vi "Read State.vi"(8 "error in (no error)":errorcluster, 11 "HECR in":refnum<class "PL SMC HECR.lvclass">) -> (0 "error out":errorcluster, 2 "state":T1, 3 "HECR out":refnum<class "PL SMC HECR.lvclass">)   [LabVIEW 2015, in "PL SMC HECR.lvclass"]
doc: "Reads device state."
uses:
  PL SMC HECR.lvclass
  <vilib>/plasmapper/PL Modbus Client/PL Modbus Client.lvclass
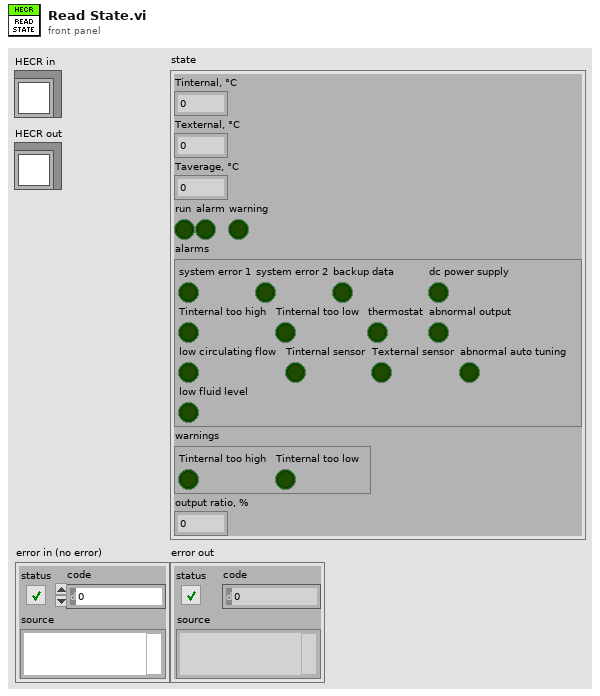
[diagram p1: front panel]
types:
  T1 = cluster{"Tinternal, °C":dbl, "Texternal, °C":dbl, "Taverage, °C":dbl, "run":bool, "alarm":bool, "warning":bool, "alarms":cluster{"system error 1":bool, "system error 2":bool, "backup data":bool, "dc power supply":bool, "Tinternal too high":bool, "Tinternal too low":bool, "thermostat":bool, "abnormal output":bool, "low circulating flow":bool, "Tinternal sensor":bool, "Texternal sensor":bool, "abnormal auto tuning":bool, "low fluid level":bool}, "warnings":cluster{"Tinternal too high":bool, "Tinternal too low":bool}, "output ratio, %":dbl}
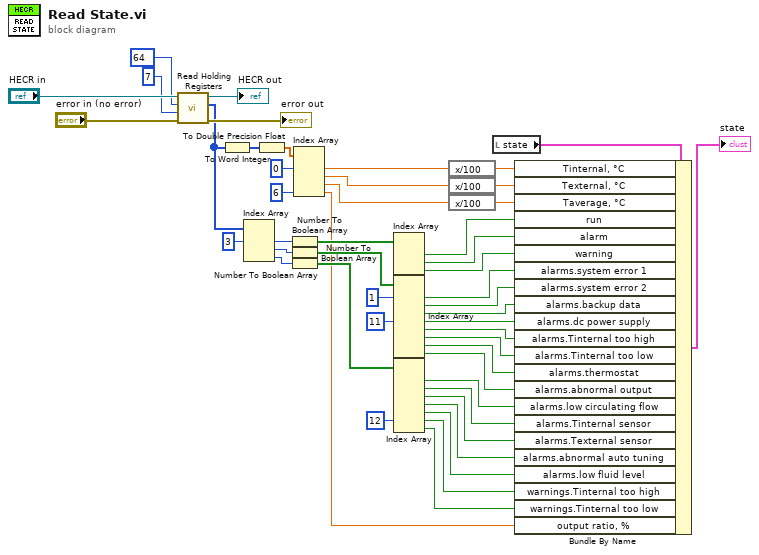
[diagram p0: block diagram]
diagram:
  n1 = call <vilib>:"Read Holding Registers.vi"("error in (no error)"="error in (no error)", "number of holding registers"=u16 7, "address"=u16 64, "MODBUS in"="HECR in") -> ("error out"=→"error out":errorcluster, "values"=w37:u16[], "MODBUS out"=→"HECR out":refnum<class "PL SMC HECR.lvclass">)  [unwired: 5 in]
  n2 = To Word Integer(number=w37) -> (16bit integer=w23:i16[])
  n3 = Index Array(array=w37, index #1=3 ("index")) -> (element #1=w35:u16, element #2=w34:u16, element #3=w33:u16)  [unwired: 2 in]
  n4 = To Double Precision Float(number=w23) -> (double precision float=w40:dbl[])
  n5 = Number To Boolean Array(number=w35) -> (Boolean array=w32:bool[])
  n6 = Number To Boolean Array(number=w34) -> (Boolean array=w31:bool[])
  n7 = Number To Boolean Array(number=w33) -> (Boolean array=w30:bool[])
  n8 = Index Array(array=w40, index #1=0 ("index"), index #4=6 ("index")) -> (element #1=w29:dbl, element #2=w28:dbl, element #3=w27:dbl, element #4=w22:dbl)  [unwired: 2 in]
  n9 = Index Array(array=w32) -> (element #1=w21:bool, element #2=w20:bool, element #3=w19:bool)  [unwired: 3 in]
  n10 = Index Array(array=w31, index #1=1 ("index"), index #4=11 ("index")) -> (element #1=w18:bool, element #2=w17:bool, element #3=w16:bool, element #4=w13:bool, element #5=w12:bool, element #6=w11:bool, element #7=w10:bool, element #8=w9:bool)  [unwired: 6 in]
  n11 = Index Array(array=w30, index #6=12 ("index")) -> (element #1=w8:bool, element #2=w7:bool, element #3=w6:bool, element #4=w5:bool, element #5=w4:bool, element #6=w2:bool, element #7=w1:bool)  [unwired: 6 in]
  n12 = expression code="x/100"(w29) -> (w26:dbl)
  n13 = expression code="x/100"(w28) -> (w25:dbl)
  n14 = expression code="x/100"(w27) -> (w24:dbl)
  n15 = local read "state"() -> (w42:T1)
  n16 = Bundle By Name(cluster=w42, "Tinternal, °C"=w26, "Texternal, °C"=w25, "Taverage, °C"=w24, "run"=w21, "alarm"=w20, "warning"=w19, "alarms.system error 1"=w18, "alarms.system error 2"=w17, "alarms.backup data"=w16, "alarms.dc power supply"=w13, "alarms.Tinternal too high"=w12, "alarms.Tinternal too low"=w11, "alarms.thermostat"=w10, "alarms.abnormal output"=w9, "alarms.low circulating flow"=w8, "alarms.Tinternal sensor"=w7, "alarms.Texternal sensor"=w6, "alarms.abnormal auto tuning"=w5, "alarms.low fluid level"=w4, "warnings.Tinternal too high"=w2, "warnings.Tinternal too low"=w1, "output ratio, %"=w22) -> (→"state":T1)
